vi "Macro Debugger.vi"(8 "Error In":errorcluster, 11 "UI control refnums":T1) -> (0 "Error Out":errorcluster, 3 "Any Error?":bool)   [LabVIEW 2012]
doc: "SciScan 1.2 160622"
uses:
  Custom Controls and Typedefs/Macro_MD_UI Control Refnums.ctl
  Custom Controls and Typedefs/Delete Button.ctl
  Custom Controls and Typedefs/Edit Button.ctl
  Custom Controls and Typedefs/Timing Estimate Cluster.ctl
  CommonResource VIs/Timing/Timing Indicator.ctl
  Custom Controls and Typedefs/Load from PSM Button.ctl
  Macro Rule/subVIs/MacroErrorsFGV_Commands.ctl
  SubVIs/FGV_MacroCore_Commands.ctl
  <vilib>/Utility/miscctls.llb/LVRowAndColumnTypeDef.ctl
  CommonResource VIs/UI Control and Indicator properties_Commands.ctl
  GFG/GFG library.lvlib
panel:
  out "Macro Command Errors":bool[](array[boolean])
  # "(hh:mm:ss)"
  # "(hh:mm:ss)"
  # "(hh:mm:ss)"
  # "(hh:mm:ss)"
  # "(hh:mm:ss)"
  # "(hh:mm:ss)"
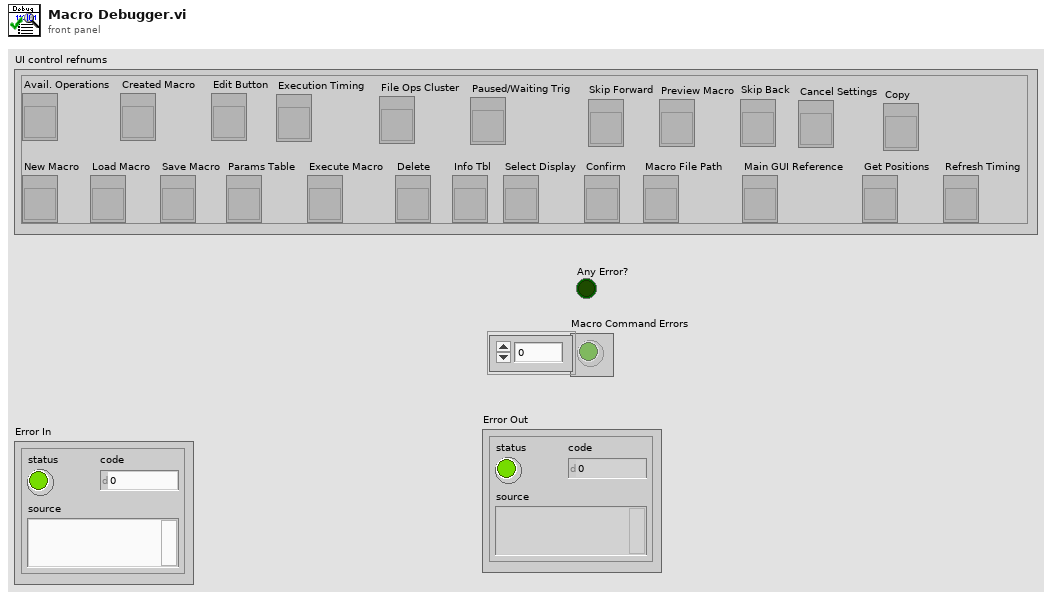
[diagram p1: front panel]
types:
  T1 = typedef "Macro_MD_UI Control Refnums.ctl" = cluster{"Avail. Operations":refnum<vi>, "Created Macro":refnum<vi>, "Load Macro":refnum<vi>, "Save Macro":refnum<vi>, "Params Table":refnum<vi>, "Delete":refnum<vi>, "Edit Button":refnum<vi>, "Execute Macro":refnum<vi>, "Info Tbl":refnum<vi>, "Execution Timing":refnum<vi>, "Select Display":refnum<vi>, "File Ops Cluster":refnum<vi>, "Paused/Waiting Trig":refnum<vi>, "Confirm":refnum<vi>, "New Macro":refnum<vi>, "Preview Macro":refnum<vi>, "Skip Forward":refnum<vi>, "Skip Back":refnum<vi>, "Macro File Path":refnum<vi>, "Main GUI Reference":refnum<vi>, "Cancel Settings":refnum<vi>, "Get Positions":refnum<vi>, "Copy":refnum<vi>, "Refresh Timing":refnum<vi>}
  T2 = typedef "FGV_MacroCore_Commands.ctl" = enum16{"Initialize", "Get Array", "Load macro from file", "Insert Item", "Insert at End", "Edit Parameter String", "Delete instruction", "Move Items", "Save", "SaveAs", "UpdateInfoTable", "Edit Settings File", "New Macro", "Read Temp File", "Delete Multiple"}
  T3 = typedef "MacroErrorsFGV_Commands.ctl" = enum16{"Initialize", "Get Error Array", "Set Error Array"}
  T4 = typedef "LVRowAndColumnTypeDef.ctl" = cluster{"Row":i32, "Column":i32}
  T5 = typedef "Macro Error Cluster.ctl" = cluster{"Error?":bool, "Description":string, "Warning?":bool}
  T6 = typedef "UI Control and Indicator properties_Commands.ctl" = enum16{"Enable", "Disable", "Disable and Grey", "Make Visible", "Make Invisible"}
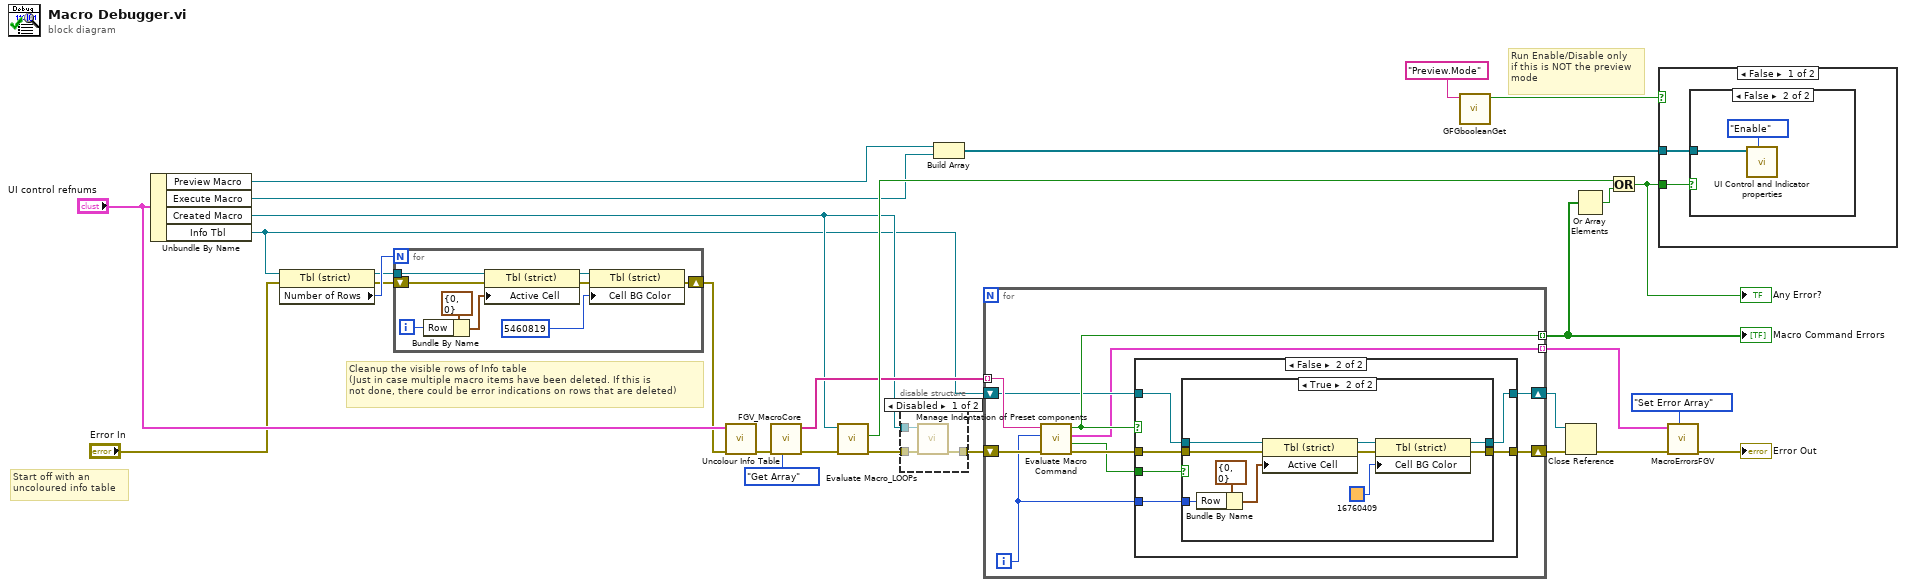
[diagram p0: block diagram]
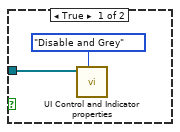
[diagram p3: hidden frame]
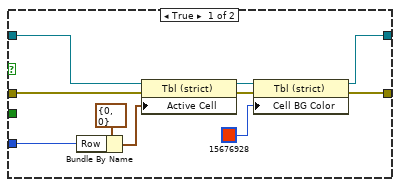
[diagram p5: hidden frame]
diagram:
  # "Cleanup the visible rows of Info table\n(Just in case multiple macro items have been deleted. If this is \nnot done, there could be error indications on rows that are deleted)"
  # "Run Enable/Disable only\nif this is NOT the preview\nmode"
  # "Start off with an \nuncoloured info table"
  n1 = Unbundle By Name("UI control refnums") -> ("Preview Macro"=w14:refnum<vi>, "Execute Macro"=w13:refnum<vi>, "Created Macro"=w7:refnum<vi>, "Info Tbl"=w6:refnum<vi>)
  n2 = property class="Tbl (strict)"(reference=w6, error in="Error In") -> (reference out=w4:refnum<vi>, error out=w2:errorcluster, "Number of Rows"=w5:u32)
  n3 = for {
    N: w5 -> [_]
    tunnel: w4 -> [w34]
    shift-right: [w32] -> w1
    shift-left: w2 -> [w31]
    i -> [w33]
    n4 = Bundle By Name(cluster=T4 {"Row"=0, "Column"=0} ("Active Cell:Active Cell"), "Row"=w33) -> (w37:T4)
    n5 = property class="Tbl (strict)"(reference=w34, error in=w31, "Active Cell"=w37) -> (reference out=w36:refnum<vi>, error out=w35:errorcluster)
    n6 = property class="Tbl (strict)"(reference=w36, error in=w35, "Cell BG Color"=u32 5460819 ("Active Cell:Cell Background Color")) -> (error out=w32:errorcluster)  [unwired: 1 out]
  }
  n7 = call "Uncolour Info Table.vi"("Error In"=w1, "UI control refnums"="UI control refnums") -> ("Error Out"=w16:errorcluster)  [unwired: 9 in]
  n8 = call "FGV_MacroCore.vi"("MacroFGV_Commands"=FGV_MacroCore_Commands."Get Array", "Error In"=w16) -> ("Error Out"=w15:errorcluster, "Macro String Array"=w19:string[])  [unwired: 5 in, 3 out]
  n9 = call "Evaluate Macro_LOOPs.vi"("Error In"=w15, "Tree Refnum IN"=w7) -> ("Error Out"=w9:errorcluster, "Macro Error"=w27:bool)  [unwired: 8 in]
  n10 = disable-structure shown="Disabled" {
    disable-tunnel: w9 -> [w41 w42]
    disable-tunnel: [w40 w42] -> w8
    disable-tunnel: w7 -> [w39 _]
    frame Disabled {
      n11 = call "Manage Indentation of Preset components.vi"("error in (no error)"=w41, "Tree Refnum"=w39) -> ("error out"=w40:errorcluster)  [unwired: 9 in]
    }
    frame Enabled {
    }
  }
  n12 = Build Array(w14, w13) -> (w12:refnum<vi>[])
  n13 = for {
    tunnel: w19 -> [w51] mode=indexing
    tunnel: [w50] -> w29 mode=indexing
    shift-right: [w46] -> w26
    shift-left: w8 -> [w52]
    shift-right: [w47] -> w25
    shift-left: w6 -> [w49]
    tunnel: [w45] -> w23 mode=indexing
    i -> [w43]
    n14 = call "Evaluate Macro Command.vi"("Error In"=w52, "Cmd Index"=w43, "Macro Command String IN"=w51) -> ("Error Out"=w48:errorcluster, "Warning?"=w44:bool, "Macro Error Cluster"=w45:T5, "Error in Command?"=w50:bool)  [unwired: 5 in]
    n15 = case shown="False" w50 {
      tunnel: w49 -> [w62 w65]
      tunnel: w43 -> [w60 w63]
      tunnel: w48 -> [w58 w67]
      tunnel: [w54 w64] -> w47
      tunnel: [w53 w66] -> w46
      tunnel: w44 -> [_ w68]
      frame True {
        n16 = Bundle By Name(cluster=T4 {"Row"=0, "Column"=0} ("Active Cell:Active Cell"), "Row"=w60) -> (w59:T4)
        n17 = property class="Tbl (strict)"(reference=w62, error in=w58, "Active Cell"=w59) -> (reference out=w57:refnum<vi>, error out=w56:errorcluster)
        n18 = property class="Tbl (strict)"(reference=w57, error in=w56, "Cell BG Color"=u32 15676928) -> (reference out=w54:refnum<vi>, error out=w53:errorcluster)
      }
      frame False {
        n19 = case shown="True" w68 {
          tunnel: w67 -> [w69 w75]
          tunnel: [w69 w74] -> w66
          tunnel: w65 -> [w70 w73]
          tunnel: [w70 w72] -> w64
          tunnel: w63 -> [_ w71]
          frame False {
          }
          frame True {
            n20 = Bundle By Name(cluster=T4 {"Row"=0, "Column"=0} ("Active Cell:Active Cell"), "Row"=w71) -> (w79:T4)
            n21 = property class="Tbl (strict)"(reference=w73, error in=w75, "Active Cell"=w79) -> (reference out=w78:refnum<vi>, error out=w77:errorcluster)
            n22 = property class="Tbl (strict)"(reference=w78, error in=w77, "Cell BG Color"=u32 16760409) -> (reference out=w72:refnum<vi>, error out=w74:errorcluster)
          }
        }
      }
    }
  }
  "Macro Command Errors" <- w29
  n23 = call "GFGbooleanGet.vi"("Variable Name in"="Preview.Mode") -> ("Boolean Value OUT"=w10:bool)  [unwired: 9 in, 1 out]
  n24 = Close Reference(reference=w25, error in (no error)=w26) -> (error out=w24:errorcluster)
  n25 = Or Array Elements(Boolean array=w29) -> (logical OR=w28:bool)
  n26 = Or(x=w27, y=w28) -> (x .or. y?=w21:bool)
  "Any Error?" <- w21
  n27 = case shown="False" w10 {
    tunnel: w21 -> [w82 _]
    tunnel: w12 -> [w81 _]
    frame False {
      n28 = case shown="False" w82 {
        tunnel: w81 -> [w83 w85]
        frame True {
          n29 = call "UI Control and Indicator properties.vi"("Enable Command"=UI_Control_and_Indicator_properties_Commands."Disable and Grey", "Control Refnums"=w83) -> ()  [unwired: 9 in, 1 out]
        }
        frame False {
          n30 = call "UI Control and Indicator properties.vi"("Enable Command"=UI_Control_and_Indicator_properties_Commands."Enable", "Control Refnums"=w85) -> ()  [unwired: 9 in, 1 out]
        }
      }
    }
    frame True {
    }
  }
  n31 = call "MacroErrorsFGV.vi"("MacroErrorsFGV_Commands"=MacroErrorsFGV_Commands."Set Error Array", "Error In"=w24, "Error Array IN"=w23) -> ("Error Out"=→"Error Out":errorcluster)  [unwired: 7 in, 1 out]
